vi "wpi swerve.vi"   [LabVIEW 2023]
uses:
  <vilib>/Rock Robotics/WPI/Joystick/XBox Axes Indexer.ctl
  <vilib>/Rock Robotics/WPI/ThirdParty/JAS_Junk/TrajLib/Rotation2d_GetCos.vi
  <vilib>/Rock Robotics/WPI/ThirdParty/JAS_Junk/TrajLib/Rotation2d_GetSin.vi
  <vilib>/Rock Robotics/WPI/ThirdParty/JAS_Junk/TrajLib/ChassisSpeeds_New.vi
  <vilib>/Rock Robotics/WPI/Utilities/WPI_GetSetVariantRefNum.vi
  <vilib>/Rock Robotics/WPI/ThirdParty/JAS_Junk/TrajLib/Trajectory_Library.lvlib
types:
  T1 = typedef "XBox Axes Indexer.ctl" = enum16{"Left X", "Left Y", "Left Trigger", "Right Trigger", "Right X", "Right Y"}
  T2 = typedef "ADIS16470 Device Reference.ctl" = cluster{"DevStatus":errorcluster, "Hardware Config":T3, "Calibration Complete":refnum<notifier>, "Status Reference":refnum<data-value>, "Data Reference":refnum<data-value>, "Sychronous Process VI":T7, "Cmd FIFO":refnum<k33>, "Source":T8, "Data FIFO":refnum<k33>, "Calibration Time (ms)":u32, "Data Reference":refnum<data-value>}
  T3 = typedef "ADIS16470 Hardware Configuration.ctl" = cluster{"SPI Clock Rate (Hz)":dbl, "IMU SPI Mode (3)":T4, "IMU Reset Pin":T5, "IMU SPI Bus":T6, "IMU Data Ready Pin":T5, "Stall Config":cluster{"Pow2BytesPerRead":u8, "StallTicks":u16, "CsToSclkTicks":u8}}
  T4 = typedef "WPI_SPIMode.ctl" = enum16{"Mode 0 (Clk Idle Low,Sample on Leading)", "Mode 1 (Clk Idle Low,Sample on Trailing)", "Mode 2 (Clk Idle High,Sample on Leading)", "Mode 3 (Clk Idle High,Sample on Trailing)"}
  T5 = typedef "FPGA_DIOChannel.ctl" = enum8{"DIO 0", "DIO 1", "DIO 2", "DIO 3", "DIO 4", "DIO 5", "DIO 6", "DIO 7", "DIO 8", "DIO 9", "DIO MXP 0", "DIO MXP 1", "DIO MXP 2", "DIO MXP 3", "DIO MXP 4", "DIO MXP 5", "DIO MXP 6", "DIO MXP 7", "DIO MXP 8", "DIO MXP 9", "DIO MXP 10", "DIO MXP 11", "DIO MXP 12", "DIO MXP 13", "DIO MXP 14", "DIO MXP 15", "SPI Port CS1", "SPI Port CS2", "SPI Port CS3", "SPI Port MISO", "SPI Port MOSI", "Invalid"}
  T6 = typedef "spi_bus.ctl" = enum16{"SPI On-Board, CS0", "SPI On-Board, CS1", "SPI On-Board, CS2", "SPI On-Board, CS3", "SPI MXP", "Invalid"}
  T7 = typedef "ADIS16470 Process.ctl" = refnum<vi>
  T8 = typedef "FPGA_CounterEncoderSourceConvertionLVSourceType.ctl" = cluster{"DevStatus":errorcluster, "AnalogTriggerMode?":bool, "DigitalMode":cluster{"DIO Channel":T9}, "AnalogTriggerMode":cluster{"AnalogTriggerIndex":T10, "OutputType":T11}}
  T9 = typedef "FPGA_DIODigitalSourceChannel.ctl" = enum8{"DIO 0", "DIO 1", "DIO 2", "DIO 3", "DIO 4", "DIO 5", "DIO 6", "DIO 7", "DIO 8", "DIO 9", "DIO MXP 0", "DIO MXP 1", "DIO MXP 2", "DIO MXP 3", "DIO MXP 4", "DIO MXP 5", "DIO MXP 6", "DIO MXP 7", "DIO MXP 8", "DIO MXP 9", "DIO MXP 10", "DIO MXP 11", "DIO MXP 12", "DIO MXP 13", "DIO MXP 14", "DIO MXP 15", "SPI Port CS1", "SPI Port CS2", "SPI Port CS3", "SPI Port MISO", "SPI Port MOSI", "Disabled"}
  T10 = typedef "FPGA_AnalogTriggerIndex.ctl" = enum8{"Trig 0", "Trig 1", "Trig 2", "Trig 3", "Trig 4", "Trig 5", "Trig 6", "Trig 7", "Invalid"}
  T11 = typedef "FPGA_AnalogTriggerOutType.ctl" = enum16{"InWindow", "TriggerState", "Rising", "Falling"}
  T12 = typedef "ADIS16470 Data.ctl" = cluster{"XAngle":dbl, "YAngle":dbl, "ZAngle":dbl}
  T13 = typedef "WPI_JoystickDevRef.ctl" = cluster{"Device":T14}
  T14 = typedef "WPI_JoystickDeviceEnum.ctl" = enum16{"USB 0", "USB 1", "USB 2", "USB 3", "USB 4", "USB 5"}
  T15 = typedef "Trajectory_Library.lvlib/ROTATION2D.ctl" = cluster{"VALUE":dbl, "COS":dbl, "SIN":dbl}
  T16 = typedef "Trajectory_Library.lvlib/CHASSIS_SPEEDS.ctl" = cluster{"vX":dbl, "vY":dbl, "vOmega":dbl}
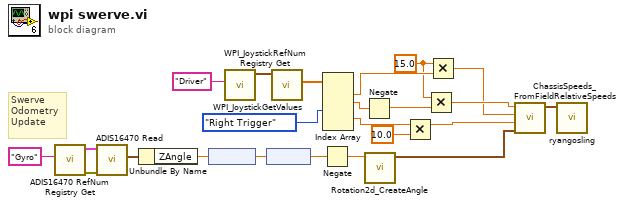
[diagram p0: block diagram]
diagram:
  w6 = 15.0 ("x")
  # "Swerve\nOdometry\nUpdate"
  n1 = call <vilib>:"ADIS16470 RefNum Registry Get.vi"("refnum name"="Gyro") -> ("error out"=w15:errorcluster, "ADIS16470DevRef out"=w16:T2)  [unwired: 9 in]
  n2 = call <vilib>:"ADIS16470 Read.vi"("error in (no error)"=w15, "ADIS16470DevRef"=w16) -> ("ADIS16470 Value"=w17:T12)  [unwired: 6 in, 3 out]
  n3 = Unbundle By Name(w17) -> ("ZAngle"=w22:dbl)
  n4 = node(w22) -> (w12:dbl[unit])
  n5 = call <vilib>:"WPI_JoystickRefNum Registry Get.vi"("refnum name"="Driver") -> ("JoystickDevRef"=w20:T13)  [unwired: 1 in, 9 out]
  n6 = node(w12) -> (w11:dbl)
  n7 = call <vilib>:"WPI_JoystickGetValues.vi"("JoystickDevRef"=w20) -> ("Axes"=w18:dbl[])  [unwired: 6 in, 4 out]
  n8 = Negate(x=w11) -> (-x=w10:dbl)
  n9 = Index Array(array=w18, index #3=XBox_Axes_Indexer."Right Trigger" ("XBox Axes")) -> (element #1=w7:dbl, element #2=w13:dbl, element #4=w3:dbl)  [unwired: 4 in, 2 out]
  n10 = Negate(x=w13) -> (-x=w8:dbl)
  n11 = call <vilib>:"Rotation2d_CreateAngle.vi"("Angle"=w10) -> ("ROTATION"=w9:T15)  [unwired: 10 in]
  n12 = Multiply(x=w3, y=10.0) -> (x*y=w2:dbl)
  n13 = Multiply(x=w6, y=w8) -> (x*y=w5:dbl)
  n14 = Multiply(x=w6, y=w7) -> (x*y=w4:dbl)
  n15 = call <vilib>:"ChassisSpeeds_FromFieldRelativeSpeeds.vi"("RobotAngle"=w9, "Omega"=w2, "vY"=w4, "vX"=w5) -> ("CHASSIS"=w23:T16)  [unwired: 7 in]
  n16 = call "ryangosling.vi"("CHASSIS"=w23) -> ()  [unwired: 9 in, 2 out]
